vi "Close Hardware.vi"(8 "error in (no error)":errorcluster, 11 "Inst.Framework-Template in":refnum<class "Inst.Framework-Template.lvclass">) -> (0 "error out":errorcluster, 3 "Inst.Framework-Template out":refnum<class "Inst.Framework-Template.lvclass">)   [LabVIEW 2019, in "Inst.Framework-Template.lvclass"]
uses:
  Inst.Framework-Template.lvclass
  Inst.Framework-Template.lvclass/Inst.Framework-Template.ctl
  <userlib>/LevyLab/Instrument Framework/Instrument Types/VSource/Instrument.VSource.lvclass
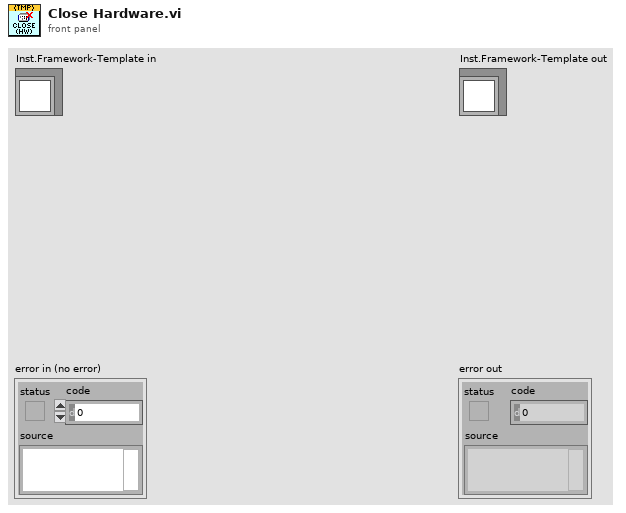
[diagram p1: front panel]
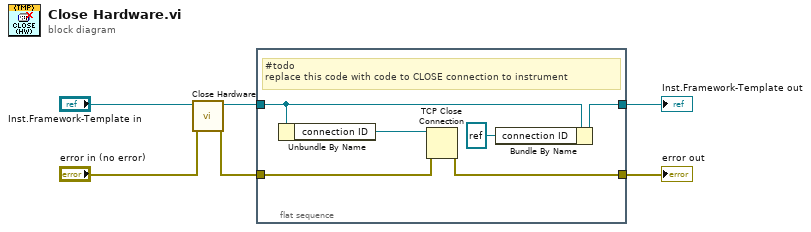
[diagram p0: block diagram]
diagram:
  n1 = call-parent "Close Hardware.vi"("error in (no error)"="error in (no error)", "Instrument in"="Inst.Framework-Template in") -> ("error out"=w4:errorcluster, "Instrument out"=w2:refnum<class "Inst.Framework-Template.lvclass">)  [unwired: 8 in]
  n2 = flat-sequence {
    tunnel: w4 -> [w11]
    tunnel: [w10] -> w3
    tunnel: w2 -> [w8]
    tunnel: [w7] -> w1
    frame #0 {
      # "#todo\nreplace this code with code to CLOSE connection to instrument"
      n3 = Unbundle By Name(w8) -> ("connection ID"=w12:refnum<k5>)
      n4 = TCP Close Connection(connection ID=w12, error in (no error)=w11) -> (error out=w10:errorcluster)  [unwired: 1 in, 1 out]
      n5 = Bundle By Name(cluster=w8, "connection ID"=refnum<k5> refnum) -> (w7:refnum<class "Inst.Framework-Template.lvclass">)
    }
  }
  "error out" <- w3
  "Inst.Framework-Template out" <- w1
